vi "Capture@PatternMatchOne(Fast)__Parameter.vi"(1 "ParamterIn":string) -> (0 "ParamterOut":string)   [LabVIEW 2020]
uses:
  MainFrame/Global.vi
panel:
  out "Image":T1(plugin-control)
  in  "Picture":string(combo)
  in  "AngleEnd":string(combo)
  in  "AngleStart":string(combo)
  in  "Score":string(combo)
  in  "Point":string(combo)
  in  "CamName":string(combo)
  in  "Confirm":bool
  # "Capture@PatternMatch/GeoMatch $Capture,$Picture,$Score,$Point(,$Angle=XX~XX)"
  # "Angle="
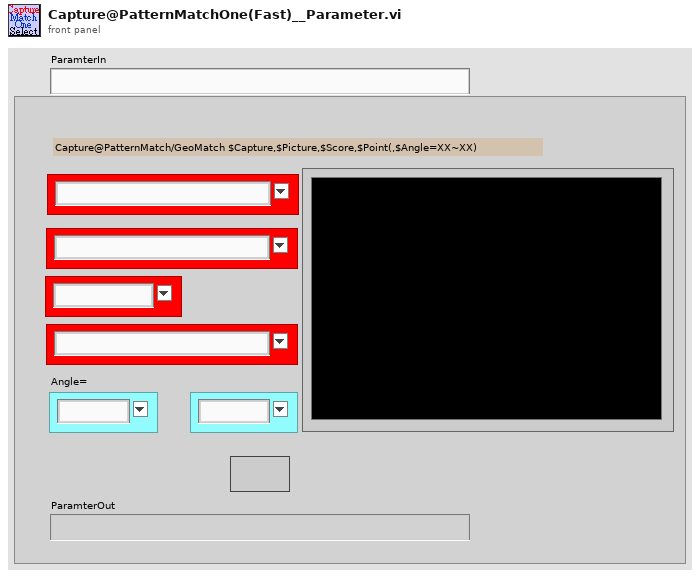
[diagram p1: front panel]
types:
  T1 = typedef "IMAQ Image.ctl" = refnum<image>
  T2 = enum16{"Get", "UpdatePointS", "Init", "UpdateIndex", "GetCurrent&Index+1", "GetWithIndex", "ChkLast", "GetCurrent"}
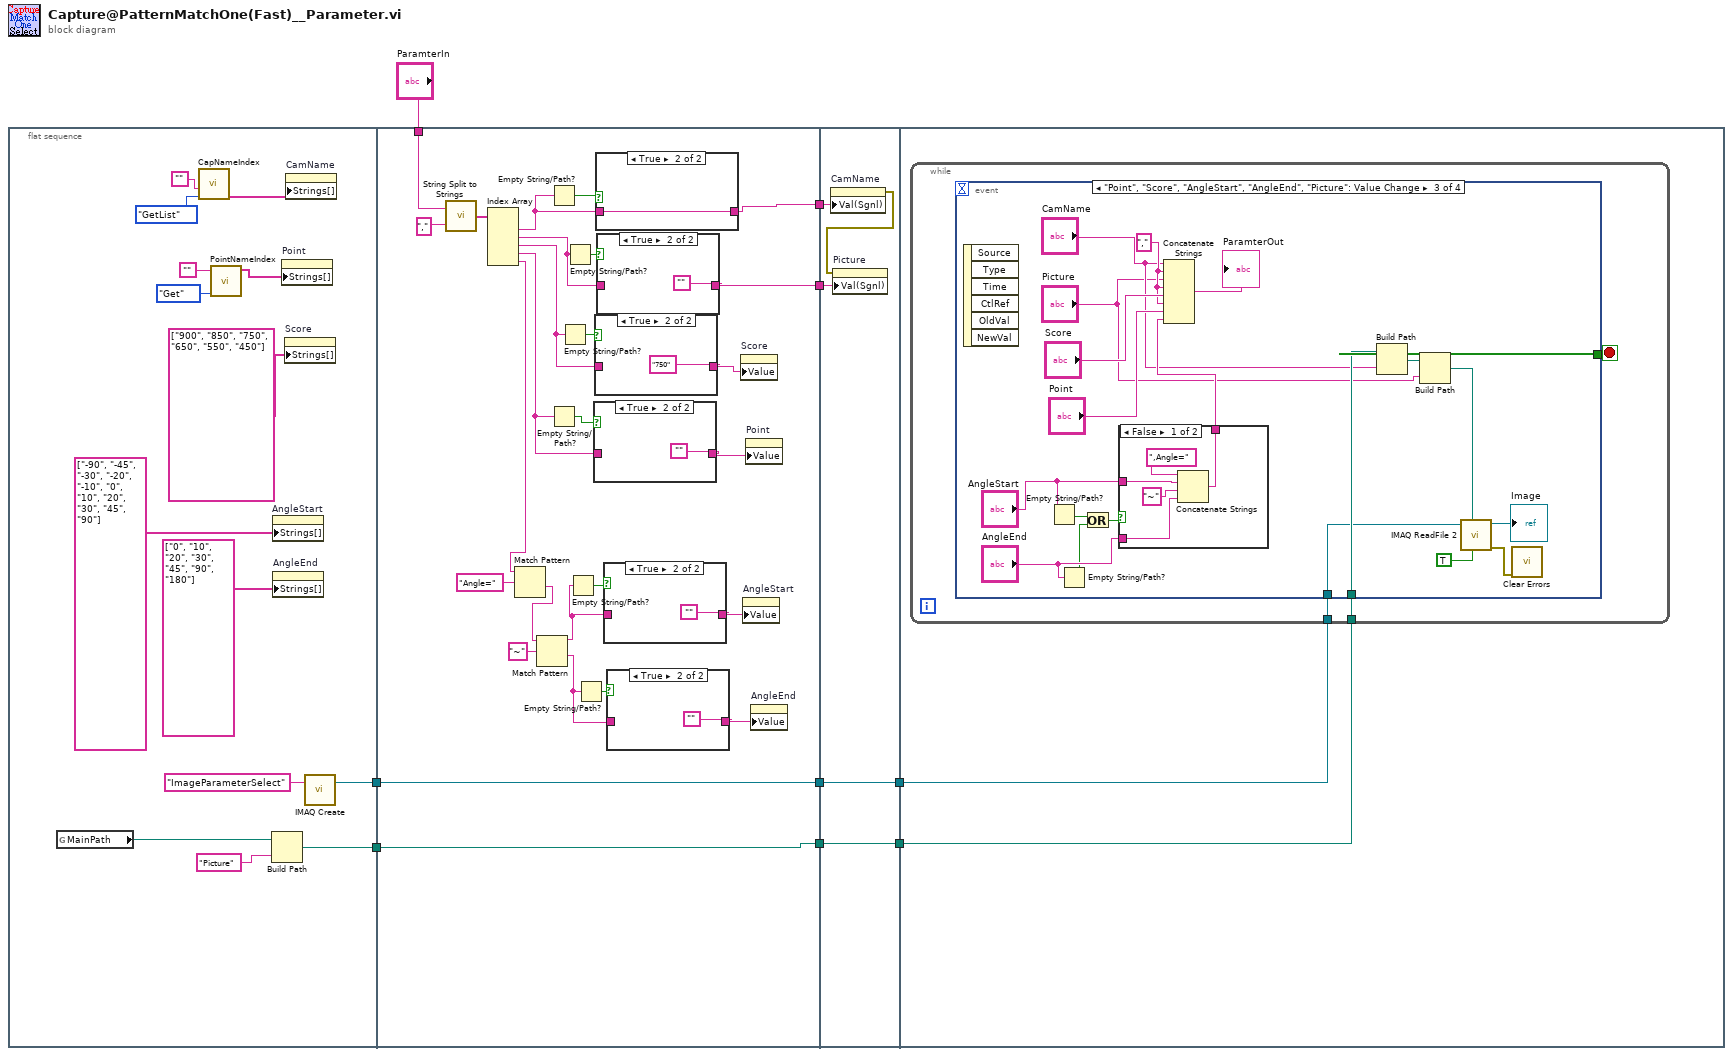
[diagram p0: block diagram]
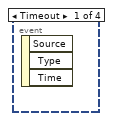
[diagram p8: hidden frame]
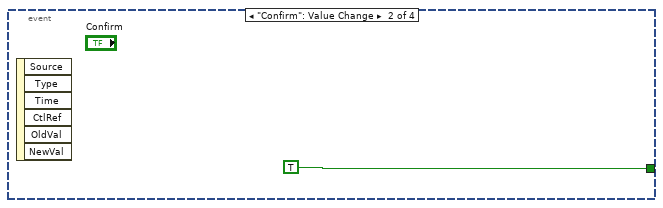
[diagram p9: hidden frame]
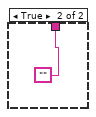
[diagram p10: hidden frame]
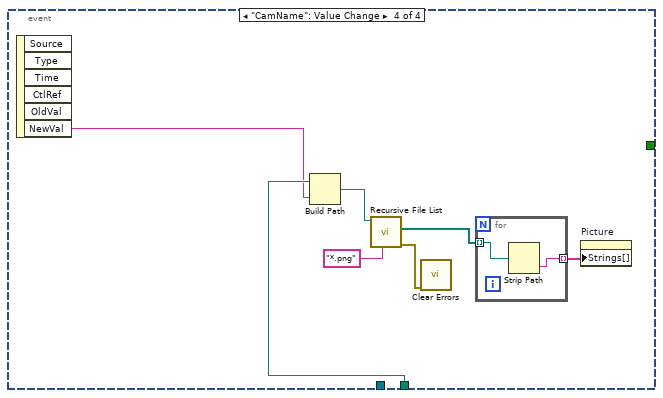
[diagram p11: hidden frame]
diagram:
  n1 = flat-sequence {
    tunnel: [w14] -> w8
    tunnel: [w12] -> w3
    tunnel: "ParamterIn" -> [w48]
    tunnel: w8 -> [w29]
    tunnel: [w29] -> w7
    tunnel: [w27] -> w4
    tunnel: w3 -> [w27]
    tunnel: [w25] -> w2
    tunnel: [w24] -> w1
    tunnel: w7 -> [w67]
    tunnel: [w67] -> w6
    tunnel: [w66] -> w5
    tunnel: w4 -> [w66]
    tunnel: w2 -> [w65]
    tunnel: w1 -> [w64]
    tunnel: w6 -> [w69]
    tunnel: w5 -> [w68]
    frame #0 {
      n2 = global read "Global.vi" "MainPath"() -> (w10:path)
      n3 = call "CapNameIndex.vi"("OP"=enum16{"AddCam", "GetIndex", "Init", "GetList"}."GetList", "CamName"="") -> ("DeviceList"=w22:string[])  [unwired: 2 in, 3 out]
      n4 = call "PointNameIndex.vi"("OP"=T2."Get", "PointName"="") -> ("PointNameList"=w18:string[])  [unwired: 4 in, 5 out]
      n5 = Build Path(base path=w10, name or relative path="Picture") -> (appended path=w12:path)
      n6 = property on="AngleStart" class="CmbBox"("Strings[]"=string[] ["-90", "-45", "-30", "-20", "-10", "0", "10", "20", "30", "45", "90"] ("Strings []")) -> ()  [unwired: 2 in, 2 out]
      n7 = property on="AngleEnd" class="CmbBox"("Strings[]"=string[] ["0", "10", "20", "30", "45", "90", "180"] ("Strings []")) -> ()  [unwired: 2 in, 2 out]
      n8 = property on="Point" class="CmbBox"("Strings[]"=w18) -> ()  [unwired: 2 in, 2 out]
      n9 = property on="Score" class="CmbBox"("Strings[]"=string[] ["900", "850", "750", "650", "550", "450"] ("Strings []")) -> ()  [unwired: 2 in, 2 out]
      n10 = property on="CamName" class="CmbBox"("Strings[]"=w22) -> ()  [unwired: 2 in, 2 out]
      n11 = call "IMAQ Create"("Image Name"="ImageParameterSelect") -> ("New Image"=w14:T1)  [unwired: 4 in, 1 out]
    }
    frame #1 {
      n12 = call "String Split to Strings.vi"("search string/char (-)"=",", "String"=w48) -> ("Array"=w50:string[])
      n13 = Index Array(array=w50) -> (element #1=w28:string, element #2=w40:string, element #3=w43:string, element #4=w45:string, element #5=w39:string)  [unwired: 5 in]
      n14 = Match Pattern(string=w39, regular expression="Angle=") -> (after substring=w37:string)  [unwired: 1 in, 3 out]
      n15 = Match Pattern(string=w37, regular expression="~") -> (before substring=w34:string, after substring=w32:string)  [unwired: 1 in, 2 out]
      n16 = Empty String/Path?(string/path=w28) -> (empty?=w47:bool)
      n17 = Empty String/Path?(string/path=w45) -> (empty?=w46:bool)
      n18 = Empty String/Path?(string/path=w43) -> (empty?=w44:bool)
      n19 = Empty String/Path?(string/path=w40) -> (empty?=w41:bool)
      n20 = Empty String/Path?(string/path=w34) -> (empty?=w35:bool)
      n21 = Empty String/Path?(string/path=w32) -> (empty?=w33:bool)
      n22 = case shown="True" w46 {
        tunnel: [w59 ""] -> w26
        tunnel: w45 -> [w59 _]
        frame False {
        }
        frame True {
        }
      }
      n23 = case shown="True" w44 {
        tunnel: [w57 "750"] -> w42
        tunnel: w43 -> [w57 _]
        frame False {
        }
        frame True {
        }
      }
      n24 = case shown="True" w47 {
        tunnel: w28 -> [w61 w62]
        tunnel: [w61 w62] -> w24
        frame False {
        }
        frame True {
        }
      }
      n25 = case shown="True" w41 {
        tunnel: [w55 ""] -> w25
        tunnel: w40 -> [w55 _]
        frame False {
        }
        frame True {
        }
      }
      n26 = case shown="True" w35 {
        tunnel: [w53 ""] -> w31
        tunnel: w34 -> [w53 _]
        frame False {
        }
        frame True {
        }
      }
      n27 = case shown="True" w33 {
        tunnel: [w51 ""] -> w30
        tunnel: w32 -> [w51 _]
        frame False {
        }
        frame True {
        }
      }
      n28 = property on="Score" class="CmbBox"("Value"=w42) -> ()  [unwired: 2 in, 2 out]
      n29 = property on="AngleStart" class="CmbBox"("Value"=w31) -> ()  [unwired: 2 in, 2 out]
      n30 = property on="Point" class="CmbBox"("Value"=w26) -> ()  [unwired: 2 in, 2 out]
      n31 = property on="AngleEnd" class="CmbBox"("Value"=w30) -> ()  [unwired: 2 in, 2 out]
    }
    frame #2 {
      n32 = property on="CamName" class="CmbBox"("Val(Sgnl)"=w64) -> (error out=w63:errorcluster)  [unwired: 2 in, 1 out]
      n33 = property on="Picture" class="CmbBox"(error in=w63, "Val(Sgnl)"=w65) -> ()  [unwired: 1 in, 2 out]
    }
    frame #3 {
      n34 = while {
        tunnel: w69 -> [w71]
        tunnel: w68 -> [w70]
        stop <- w72 stop-if-true
        n35 = event shown="[2] \"Point\", \"Score\", \"AngleStart\", \"AngleEnd\", \"Picture\": Value Change" {
          selector: _ -> [_ _ _ _]
          dyn-events: _ -> [_ _ _ _]
          timeout: _ -> [_ _ _ _]
          tunnel: [_ TRUE _ _] -> w72
          tunnel: w71 -> [_ _ w75 _]
          tunnel: w70 -> [_ _ w82 w102]
          event Timeout {
            n36 = event-data() -> ()  [unwired: 1 in, 3 out]
          }
          event "Confirm": Value Change {
            n37 = event-data() -> ()  [unwired: 1 in, 6 out]
          }
          event "Point", "Score", "AngleStart", "AngleEnd", "Picture": Value Change {
            w89 = "," ("string")
            n38 = event-data() -> ()  [unwired: 1 in, 6 out]
            n39 = Empty String/Path?(string/path="AngleStart") -> (empty?=w84:bool)
            n40 = Empty String/Path?(string/path="AngleEnd") -> (empty?=w83:bool)
            n41 = Or(x=w84, y=w83) -> (x .or. y?=w85:bool)
            n42 = case shown="False" w85 {
              tunnel: [w95 ""] -> w88
              tunnel: "AngleStart" -> [w94 _]
              tunnel: "AngleEnd" -> [w93 _]
              frame False {
                n43 = Concatenate Strings(",Angle=" ("string"), w94, "~", w93) -> (w95:string)
              }
              frame True {
              }
            }
            n44 = Concatenate Strings("CamName", w89, "Picture", w89, "Score", w89, "Point", w88) -> (→"ParamterOut":string)
            n45 = Build Path(base path=w82, name or relative path="CamName") -> (appended path=w80:path)
            n46 = Build Path(base path=w80, name or relative path="Picture") -> (appended path=w78:path)
            n47 = call "IMAQ ReadFile 2"("Use File Path Image Type"=TRUE, "File Path"=w78, "Image"=w75) -> ("error out"=w77:errorcluster, "Image Out"=→"Image":T1)  [unwired: 4 in, 3 out]
            n48 = call <vilib>:"Clear Errors.vi"("error in (no error)"=w77) -> ()  [unwired: 5 in, 2 out]
          }
          event "CamName": Value Change {
            n49 = event-data() -> ("NewVal"=w101:string)  [unwired: 1 in, 5 out]
            n50 = Build Path(base path=w102, name or relative path=w101) -> (appended path=w100:path)
            n51 = call <vilib>:"Recursive File List.vi"("pattern"="*.png", "Folder Path"=w100) -> ("error out"=w99:errorcluster, "All Files in Dir"=w104:path[])  [unwired: 5 in, 3 out]
            n52 = call <vilib>:"Clear Errors.vi"("error in (no error)"=w99) -> ()  [unwired: 5 in, 2 out]
            n53 = for {
              tunnel: w104 -> [w107] mode=indexing
              tunnel: [w106] -> w105 mode=indexing
              n54 = Strip Path(path=w107) -> (name=w106:string)  [unwired: 1 out]
            }
            n55 = property on="Picture" class="CmbBox"("Strings[]"=w105) -> ()  [unwired: 2 in, 2 out]
          }
        }
      }
    }
  }
